vi "DSF.Execution.Runtime.Plugin Manager.Query Disk.Zips.vi"(8 "error in (no error)":errorcluster, 11 "Plugin Manager in":refnum<class "DSF.Engine.Runtime.Plugin Manager.lvclass">) -> (0 "error out":errorcluster, 2 "LLB paths":path[](array[path]), 3 "Plugin Manager out":refnum<class "DSF.Engine.Runtime.Plugin Manager.lvclass">)   [LabVIEW 2017, in "DSF.Engine.lvlib" / "DSF.Engine.Runtime.Plugin Manager.lvclass"]
uses:
  DSF.Engine.Runtime.Plugin Manager.lvclass
  DSF.Engine.Runtime.Plugin Manager.lvclass/DSF.Engine.Runtime.Plugin Manager.ctl
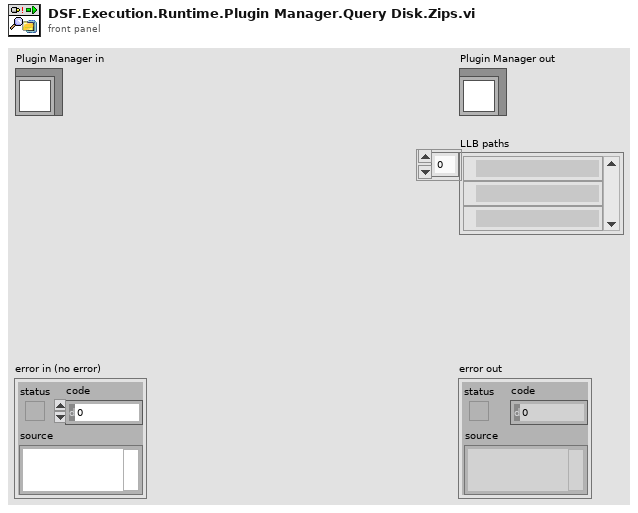
[diagram p1: front panel]
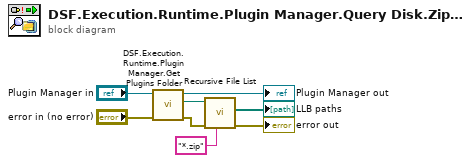
[diagram p0: block diagram]
diagram:
  n1 = call "DSF.Execution.Runtime.Plugin Manager.Get Plugins Folder.vi"("error in (no error)"="error in (no error)", "Plugin Manager in"="Plugin Manager in") -> ("error out"=w4:errorcluster, "Plugins folder"=w5:path, "Plugin Manager out"=→"Plugin Manager out":refnum<class "DSF.Engine.Runtime.Plugin Manager.lvclass">)  [unwired: 7 in]
  n2 = call <vilib>:"Recursive File List.vi"("pattern"="*.zip", "error in (no error)"=w4, "Folder Path"=w5) -> ("error out"=→"error out":errorcluster, "All Files in Dir"=→"LLB paths":path[])  [unwired: 4 in, 3 out]
